vi "programa_transmissibilidade.vi"() -> ()   [LabVIEW 2016]
uses:
  <vilib>/express/express analysis/Spectral/Block/exnSpectralBlock spectral measurements peak poly.vi
  <vilib>/express/express analysis/Spectral/Block/exnSpectralBlock spectral measurements peak DDT.vi
  <vilib>/express/express analysis/Spectral/XNode/ExpressSpectralMeasurementsBlockNode.xnode
panel:
  out "Waveform Graph":dynamicdata(graph)
  out "acel 2":dynamicdata(graph)
  out "acel 1":dynamicdata(graph)
  out "acel 3":dynamicdata(graph)
  out "acel 0":dynamicdata(graph)
  in  "stop (F)":bool
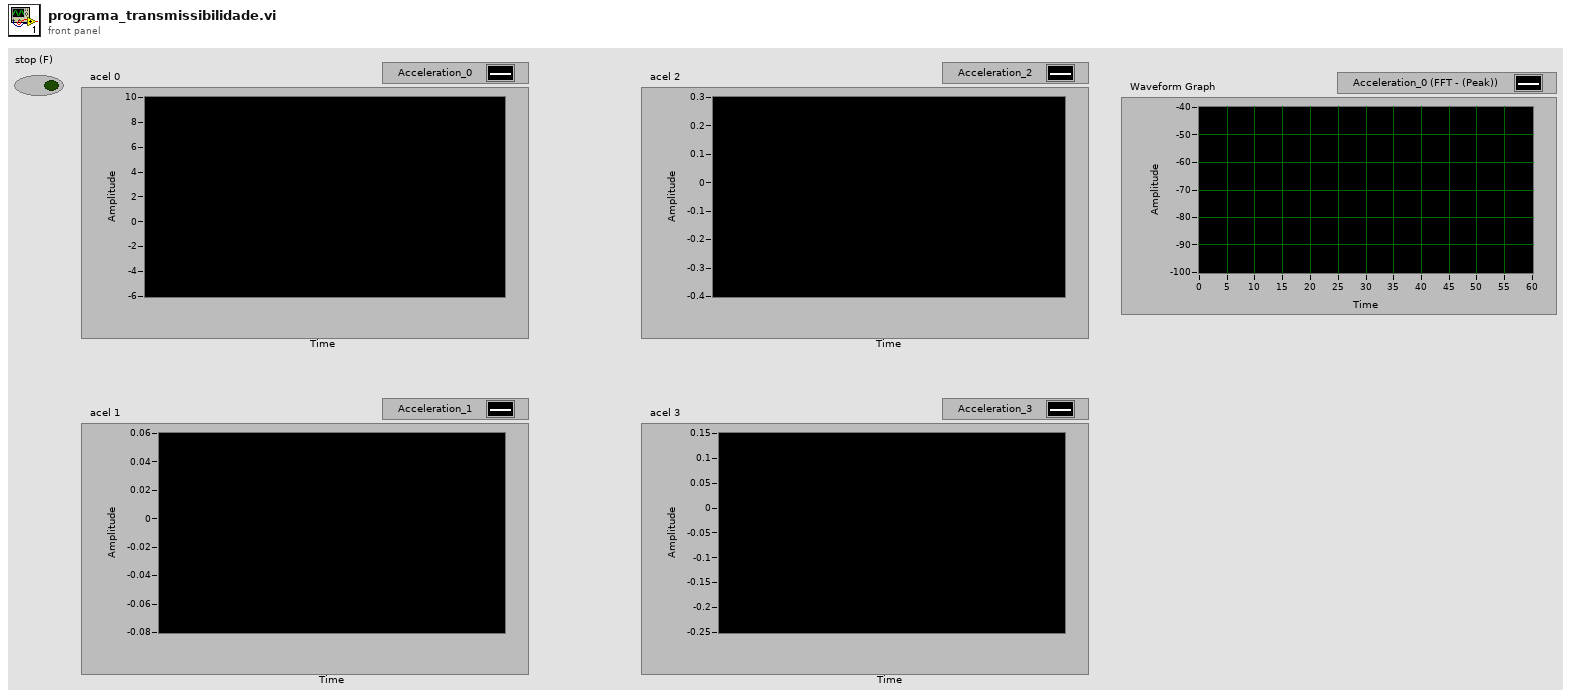
[diagram p1: front panel]
types:
  T1 = cluster{"averaging mode":u16, "weighting mode":u16, "number of averages":u32}
  T2 = cluster{"dB On (F)":bool, "unwrap phase (F)":bool, "convert to degree (F)":bool}
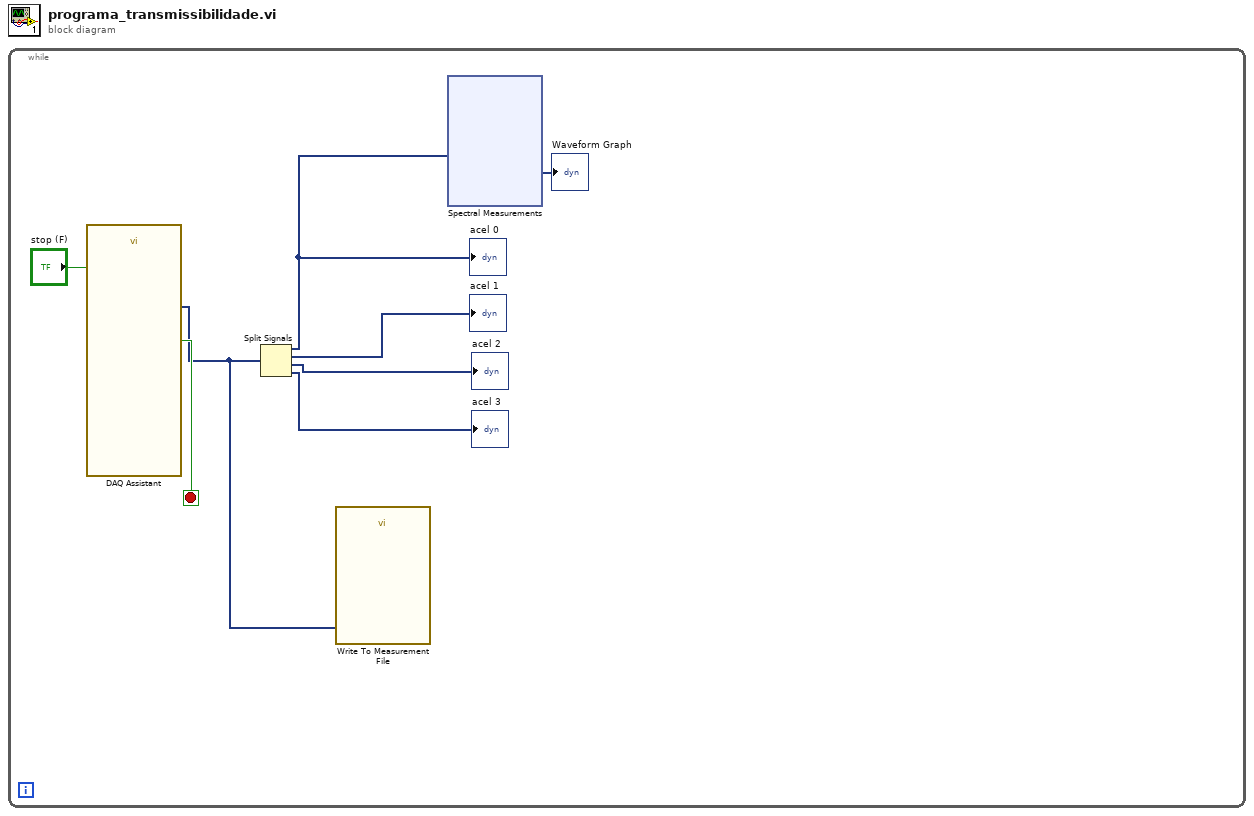
[diagram p0: block diagram]
diagram:
  n1 = while {
    stop <- w7 stop-if-true
    n2 = call "DAQ Assistant"("stop (F)"="stop (F)") -> ("data"=w1:dynamicdata, "stopped"=w7:bool)  [unwired: 15 in, 2 out]
    n3 = Split Signals(w1) -> (w3:dynamicdata, →"acel 1":dynamicdata, →"acel 2":dynamicdata, →"acel 3":dynamicdata)  [unwired: 4 in]
    "acel 0" <- w3
    n4 = call "Write To Measurement File"("Signals"=w1) -> ()  [unwired: 16 in, 3 out]
    n5 = xnode "Spectral Measurements"("Signals"=w3) -> ("FFT - (Peak)"=→"Waveform Graph":dynamicdata)  [unwired: 1 in, 2 out]
  }
